vi "Lian_Car_Specification_Converter.vi"() -> ()   [LabVIEW 2020]
panel:
  in  "Torque (lb-ft)":sgl=225.0
  out "Power (kW)":i16
  in  "Power (HP)":sgl=250.0
  out "Torque (N-m)":i16
  # "Car Specification Converter"
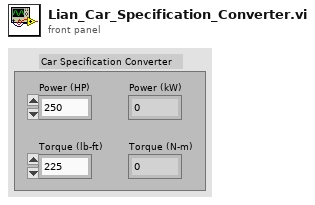
[diagram p1: front panel]
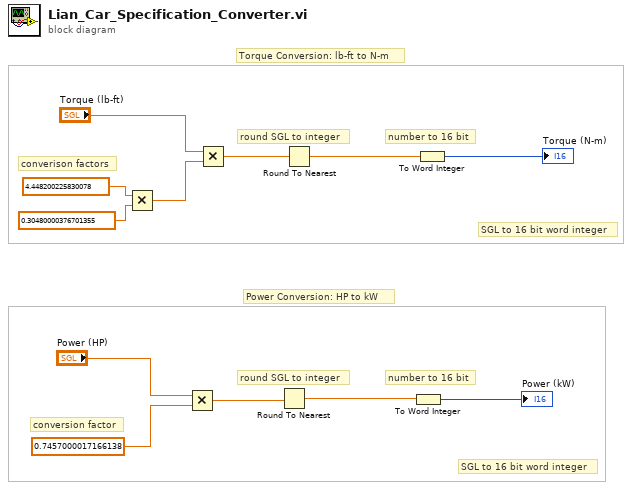
[diagram p0: block diagram]
diagram:
  # "Power Conversion: HP to kW"
  # "SGL to 16 bit word integer"
  # "number to 16 bit"
  # "round SGL to integer"
  # "conversion factor"
  # "Torque Conversion: lb-ft to N-m"
  # "SGL to 16 bit word integer"
  # "number to 16 bit"
  # "round SGL to integer"
  # "converison factors"
  n1 = Multiply(x=sgl 4.4482, y=sgl 0.3048) -> (x*y=w7:sgl)
  n2 = Multiply(x="Power (HP)", y=sgl 0.7457 ("x*y")) -> (x*y=w4:sgl)
  n3 = Multiply(x="Torque (lb-ft)", y=w7) -> (x*y=w10:sgl)
  n4 = Round To Nearest(number=w4) -> (nearest integer value=w3:sgl)
  n5 = Round To Nearest(number=w10) -> (nearest integer value=w9:sgl)
  n6 = To Word Integer(number=w3) -> (16bit integer=→"Power (kW)":i16)
  n7 = To Word Integer(number=w9) -> (16bit integer=→"Torque (N-m)":i16)
